vi "WaveGen.vi"(10 "Action":T7, 11 "Params":T6) -> (6 "Signals":T1)   [LabVIEW 2020, in "WaveGen.lvlib"]
uses:
  WaveGen.lvlib
  <extravilib>/ChannelInstances/Flex-t'WaveGen.lvlib-Gen Action.ctl'/))Channel.ctl
  Gen Action.ctl
  <extravilib>/ChannelInstances/Flex-t'WaveGen.lvlib-Gen Params.ctl'/))Channel.ctl
  Gen Params.ctl
  Timing Params.ctl
  Signal Params.ctl
  Shape.ctl
  <extravilib>/ChannelInstances/Flex-a[.](wfm(dbl))/))Channel.ctl
  <extravilib>/ChannelInstances/Flex-t'WaveGen.lvlib-Gen Params.ctl'/Event Data.ctl
  <extravilib>/ChannelInstances/Flex-t'WaveGen.lvlib-Gen Action.ctl'/Event Data.ctl
  Generate Event Data.ctl
  <extravilib>/ChannelInstances/Flex-t'WaveGen.lvlib-Gen Action.ctl'/))Channel.vi
  <extravilib>/ChannelInstances/Flex-t'WaveGen.lvlib-Gen Params.ctl'/))Channel.vi
  <extravilib>/ChannelInstances/Flex-t'WaveGen.lvlib-Gen Action.ctl'.lvlib
  <extravilib>/ChannelInstances/Flex-t'WaveGen.lvlib-Gen Params.ctl'.lvlib
  <extravilib>/ChannelInstances/Flex-a[.](wfm(dbl)).lvlib
panel:
  out "Rate":dbl
  out "Running":bool=TRUE
  out "Continuous":bool
  out "Gen Params":T2
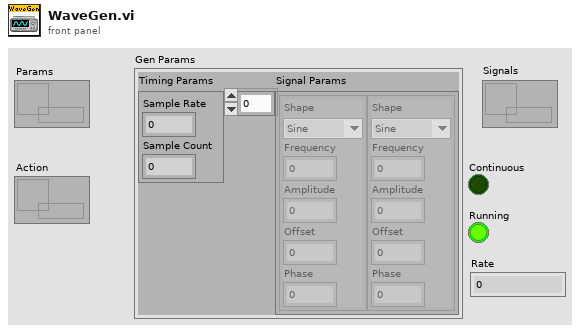
[diagram p1: front panel]
types:
  T1 = typedef "Flex-a[.](wfm(dbl)).lvlib/))Channel.ctl" = refnum<queue>
  T2 = typedef "WaveGen.lvlib/Gen Params.ctl" = cluster{"Timing Params":T3, "Signal Params":T4[]}
  T3 = typedef "WaveGen.lvlib/Timing Params.ctl" = cluster{"Sample Rate":dbl, "Sample Count":dbl}
  T4 = typedef "WaveGen.lvlib/Signal Params.ctl" = cluster{"Shape":T5, "Frequency":dbl, "Amplitude":dbl, "Offset":dbl, "Phase":dbl}
  T5 = typedef "WaveGen.lvlib/Shape.ctl" = enum16{"Sine", "Square", "Triangle", "Saw"}
  T6 = typedef "Flex-t'WaveGen.lvlib-Gen Params.ctl'.lvlib/))Channel.ctl" = refnum<queue>
  T7 = typedef "Flex-t'WaveGen.lvlib-Gen Action.ctl'.lvlib/))Channel.ctl" = refnum<queue>
  T8 = typedef "WaveGen.lvlib/Generate Event Data.ctl" = cluster{"Start":bool, "Continuous":bool}
  T9 = cluster{"Params":refnum<event-registration>, "Action":refnum<event-registration>, "Generate":refnum<event-registration>}
  T10 = typedef "WaveGen.lvlib/Gen Action.ctl" = enum16{"Run Once", "Generate", "Close", "Stop"}
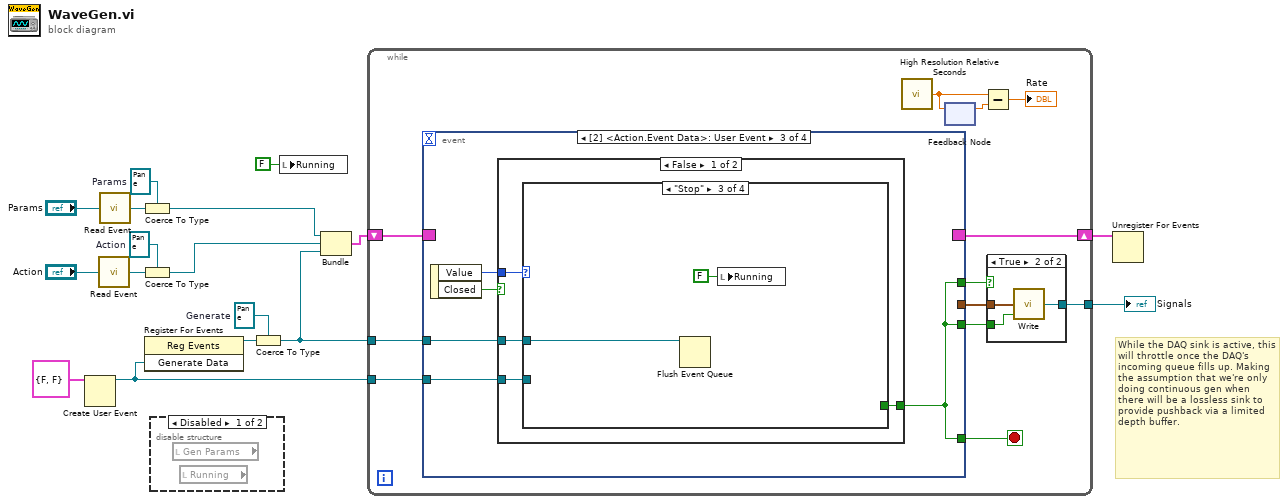
[diagram p0: block diagram]
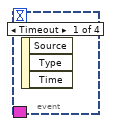
[diagram p2: hidden frame]
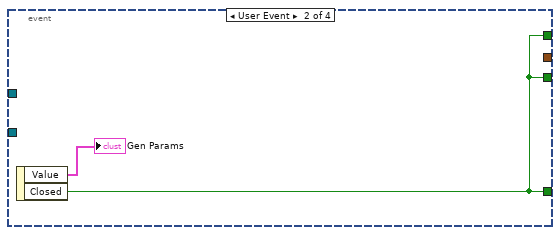
[diagram p3: hidden frame]
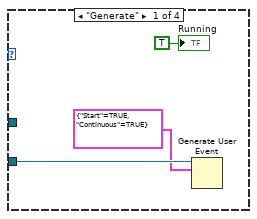
[diagram p4: hidden frame]
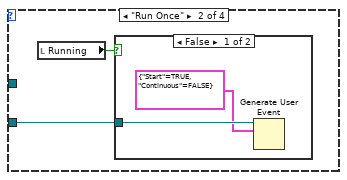
[diagram p5: hidden frame]
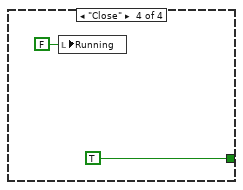
[diagram p7: hidden frame]
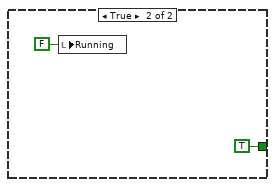
[diagram p8: hidden frame]
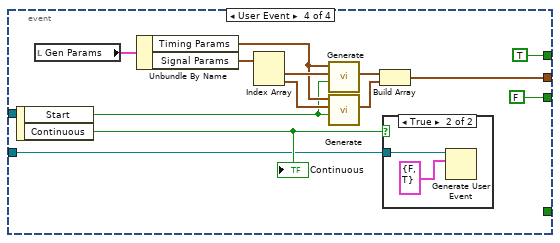
[diagram p9: hidden frame]
diagram:
  w4 = refnum<event-registration> refnum  # Generate
  w6 = refnum<event-registration> refnum  # Action
  w10 = refnum<event-registration> refnum  # Params
  # "While the DAQ sink is active, this will throttle once the DAQ's incoming queue fills up. Making the assumption that we're only doing continuous gen when there will be a lossless sink to provide pushback via a limited depth buffer."
  n1 = Create User Event(user event datatype=T8 {"Start"=FALSE, "Continuous"=FALSE} ("Generate Data")) -> (user event=w14:refnum<user-event>)  [unwired: 1 in, 1 out]
  n2 = call <extravilib>:"Read Event.vi"("FlexChannel"="Action") -> ("Event Reg"=w8:refnum<event-registration>)  [unwired: 8 in]
  n3 = call <extravilib>:"Read Event.vi"("FlexChannel"="Params") -> ("Event Reg"=w11:refnum<event-registration>)  [unwired: 8 in]
  n4 = Coerce To Type(0:w11, 1:w10) -> (2:w9:refnum<event-registration>)
  n5 = Coerce To Type(0:w8, 1:w6) -> (2:w7:refnum<event-registration>)
  n6 = register-events(w14) -> (reference out=w15:refnum<event-registration>)  [unwired: 2 in, 1 out]
  n7 = disable-structure shown="Disabled" {
    frame Disabled {
      n8 = local read "Gen Params"() -> ()  [unwired: 1 out]
      n9 = local read "Running"() -> ()  [unwired: 1 out]
    }
    frame Enabled {
    }
  }
  n10 = Coerce To Type(0:w15, 1:w4) -> (2:w13:refnum<event-registration>)
  n11 = local write "Running"(FALSE ("Running")) -> ()
  n12 = Bundle("Params"=w9, "Action"=w7, "Generate"=w13) -> (w17:T9)  [unwired: 1 in]
  n13 = while {
    shift-right: [w28] -> w2
    shift-left: w17 -> [w29]
    tunnel: w14 -> [w26]
    tunnel: w13 -> [w25]
    tunnel: [w23] -> w3
    stop <- w27 stop-if-true
    n14 = event shown="[2] <Action.Event Data>: User Event" {
      selector: w29 -> [_ _ _ _]
      dyn-events: [_ _ _ _] -> w28
      timeout: _ -> [_ _ _ _]
      tunnel: [_ w30 w33 _] -> w27
      tunnel: w26 -> [_ _ w34 w60]
      tunnel: w25 -> [_ _ w32 _]
      tunnel: [_ _ _ w56] -> w24
      tunnel: [_ w30 w33 TRUE] -> w22
      tunnel: [_ w30 w33 FALSE] -> w21
      event Timeout {
        n15 = event-data() -> ()  [unwired: 1 in, 3 out]
      }
      event User Event {
        n16 = event-data() -> ("Value"=→"Gen Params":T2, "Closed"=w30:bool)  [unwired: 1 in]
      }
      event User Event {
        n17 = event-data() -> ("Value"=w36:T10, "Closed"=w35:bool)  [unwired: 1 in]
        n18 = case shown="False" w35 {
          tunnel: w36 -> [w40 _]
          tunnel: [w39 TRUE] -> w33
          tunnel: w34 -> [w38 _]
          tunnel: w32 -> [w37 _]
          frame False {
            n19 = case shown="\"Stop\"" w40 {
              tunnel: [_ _ _ TRUE] -> w39
              tunnel: w38 -> [w43 w45 _ _]
              tunnel: w37 -> [_ _ w49 _]
              frame "Generate" {
                n20 = Generate User Event(user event=w43, event data cluster=T8 {"Start"=TRUE, "Continuous"=TRUE} ("event data")) -> ()  [unwired: 2 in, 2 out]
                "Running" <- TRUE
              }
              frame "Run Once" {
                n21 = local read "Running"() -> (w44:bool)
                n22 = case shown="False" w44 {
                  tunnel: w45 -> [w47 _]
                  frame False {
                    n23 = Generate User Event(user event=w47, event data cluster=T8 {"Start"=TRUE, "Continuous"=FALSE} ("event data")) -> ()  [unwired: 2 in, 2 out]
                  }
                  frame True {
                  }
                }
              }
              frame "Stop" {
                n24 = Flush Event Queue(0:w49) -> ()  [unwired: 5 in, 3 out]
                n25 = local write "Running"(FALSE ("Running")) -> ()
              }
              frame "Close" {
                n26 = local write "Running"(FALSE ("Running")) -> ()
              }
            }
          }
          frame True {
            n27 = local write "Running"(FALSE ("Running")) -> ()
          }
        }
      }
      event User Event {
        n28 = event-data() -> ("Start"=w57:bool, "Continuous"=w61:bool)  [unwired: 1 in]
        "Continuous" <- w61
        n29 = local read "Gen Params"() -> (w66:T2)
        n30 = Unbundle By Name(w66) -> ("Timing Params"=w63:T3, "Signal Params"=w65:T4[])
        n31 = Index Array(array=w65) -> (element #1=w64:T4, element #2=w62:T4)  [unwired: 2 in]
        n32 = call "Generate.vi"("Reset"=w57, "Gen Params"=w64, "Timing Params"=w63) -> ("signal out"=w59:waveform(dbl))  [unwired: 8 in]
        n33 = call "Generate.vi"("Reset"=w57, "Gen Params"=w62, "Timing Params"=w63) -> ("signal out"=w58:waveform(dbl))  [unwired: 8 in]
        n34 = Build Array(w59, w58) -> (w56:waveform(dbl)[])
        n35 = case shown="True" w61 {
          tunnel: w60 -> [_ w68]
          frame False {
          }
          frame True {
            n36 = Generate User Event(user event=w68, event data cluster=T8 {"Start"=FALSE, "Continuous"=TRUE} ("event data")) -> ()  [unwired: 2 in, 2 out]
          }
        }
      }
    }
    n37 = call <vilib>:"High Resolution Relative Seconds.vi"() -> ("relative seconds"=w19:dbl)
    n38 = feedback #1() -> (w20:dbl)  [unwired: 1 in]
    n39 = feedback-in #1(w19) -> ()
    n40 = Subtract(x=w19, y=w20) -> (x-y=→"Rate":dbl)
    n41 = case shown="True" w22 {
      tunnel: w24 -> [_ w71]
      tunnel: [_ w70] -> w23
      tunnel: w21 -> [_ w69]
      frame False {
      }
      frame True {
        n42 = call <extravilib>:"Write.vi"("element"=w71, "Close? (F)"=w69) -> ("channel"=w70:T1)  [unwired: 5 in, 2 out]
      }
    }
  }
  "Signals" <- w3
  n43 = Unregister For Events(event registration refnum=w2) -> ()  [unwired: 1 in, 1 out]
